vi "synnax channel retrieve keys Single.vi"(0 "Synnax Client in":refnum<class "Synnax Client.lvclass">, 5 "channel name":string, 11 "error in":errorcluster) -> (4 "Synnax Client out":refnum<class "Synnax Client.lvclass">, 6 "channel key":u32, 8 "data type":string, 10 "index key":u32, 15 "error out":errorcluster)   [LabVIEW 2026, in "synnax_lib.lvlib" / "Synnax Client.lvclass"]
doc: "SYNNAX_EXPORT int32_t synnax_channel_retrieve_keys(\n SynnaxClient client,\n const char **names,\n uint64_t name_count,\n uint32_t *out_keys,\n SynnaxError err\n);"
uses:
  Synnax Client.lvclass
  Synnax Client.lvclass/Synnax Client.ctl
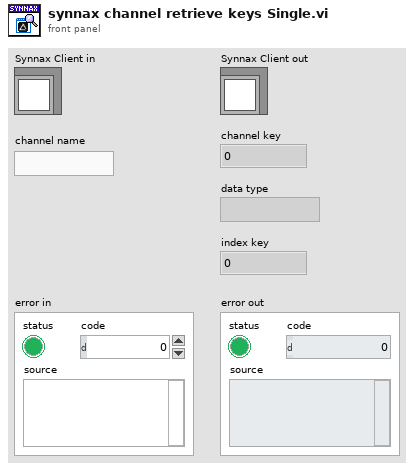
[diagram p1: front panel]
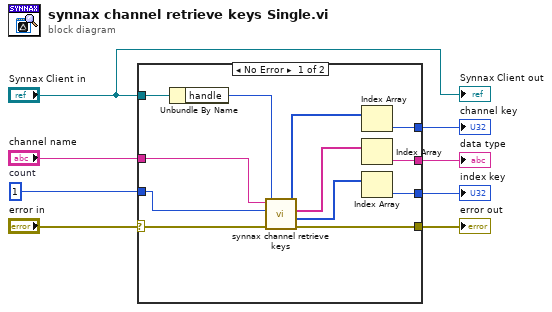
[diagram p0: block diagram]
diagram:
  w5 = u64 1  # count
  n1 = case shown="No Error" "error in" {
    selector: "error in" -> [w11 w21]
    tunnel: [w19 _] -> w8
    tunnel: "channel name" -> [w18 _]
    tunnel: "Synnax Client in" -> [w17 _]
    tunnel: w5 -> [w15 _]
    tunnel: [w13 _] -> w4
    tunnel: [w12 w21] -> w3
    tunnel: [w9 _] -> w1
    frame No Error {
      n2 = Unbundle By Name(w17) -> ("handle"=w16:u64)
      n3 = call "synnax channel retrieve keys.vi"("handle"=w16, "error in (no error)"=w11, "count"=w15, "name(s)"=w18) -> ("error out"=w12:errorcluster, "out_index_keys"=w10:u32[], "out_dtypes"=w14:string[], "out_keys"=w20:u32[])  [unwired: 4 in]
      n4 = Index Array(array=w20) -> (element=w19:u32)  [unwired: 1 in]
      n5 = Index Array(array=w14) -> (element=w13:string)  [unwired: 1 in]
      n6 = Index Array(array=w10) -> (element=w9:u32)  [unwired: 1 in]
    }
    frame Error {
    }
  }
  "channel key" <- w8
  "data type" <- w4
  "error out" <- w3
  "index key" <- w1
  "Synnax Client out" <- "Synnax Client in"
